vi "Send update actor configuration.vi"(7 "Message Priority (Normal)":T5=enum."Normal", 8 "error in (no error)":errorcluster, 10 "ActorConfiguration":T1={"GlobalConfiguration"={"DeviceFamily"="", "WriteData"=FALSE, "BufferSize_samples"=-1, "SyncDevice"=FALSE, "ExecuteInterruptRoutine"=FALSE, "InterruptRoutineTimeout_ms"=-1}, "DeviceConfiguration"={"DeviceSpecificName"="MIPI_Camera", "HardwareReference"="PXIe-Slot2", "UsedResources"=[{"ResourceLocation"="FrontFacing", "ResourceData"=variant(string "Use this Variant to store your specific resource data.\nThis will be read from and written to with the JSON parsing API.\nIn the child implementation you can use the acessors provided to convert from the specific cluster to your own device's implementation")}]}}, 11 "Message Enqueuer":refnum<class "Message Enqueuer.lvclass">) -> (0 "error out":errorcluster, 3 "Message Enqueuer out":refnum<class "Message Enqueuer.lvclass">)   [LabVIEW 2020, in "Template.lvlib" / "update actor configuration Msg.lvclass"]
doc: "This VI sends the message to an actor."
uses:
  update actor configuration Msg.lvclass
  <vilib>/ActorFramework/Message Enqueuer/Message Enqueuer.lvclass
  <vilib>/ActorFramework/Message Enqueuer/Message Priority.ctl
  template/typedefs/actor configuration.ctl
  template/typedefs/shared actor configuration.ctl
  template/typedefs/resource config/device configuration cluster.ctl
  template/typedefs/resource config/single resource cluster.ctl
  C:/Program Files/National Instruments/LabVIEW 2020/vi.lib/ActorFramework/Message/Message.lvclass
  update actor configuration Msg.lvclass/update actor configuration Msg.ctl
  <vilib>/ActorFramework/Message Enqueuer/Message Enqueuer.lvclass/Message Enqueuer.ctl
  <vilib>/ActorFramework/Message Priority Queue/Priority Enqueue.vi
  template/Template.lvclass
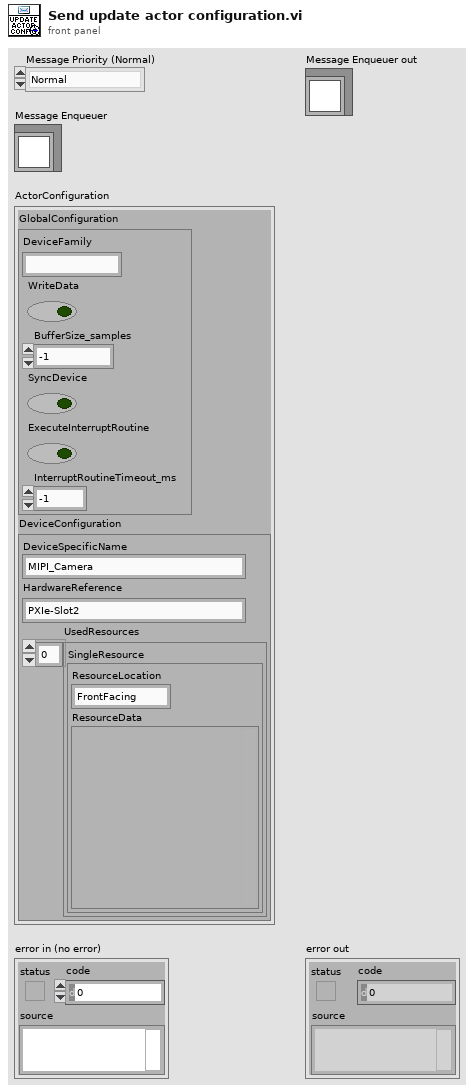
[diagram p1: front panel]
types:
  T1 = typedef "Template.lvlib/Template.lvclass/actor configuration.ctl" = cluster{"GlobalConfiguration":T2, "DeviceConfiguration":T3}
  T2 = typedef "Template.lvlib/Template.lvclass/shared actor configuration.ctl" = cluster{"DeviceFamily":string, "WriteData":bool, "BufferSize_samples":i32, "SyncDevice":bool, "ExecuteInterruptRoutine":bool, "InterruptRoutineTimeout_ms":i32}
  T3 = typedef "Template.lvlib/Template.lvclass/device configuration cluster.ctl" = cluster{"DeviceSpecificName":string, "HardwareReference":string, "UsedResources":T4[]}
  T4 = typedef "Template.lvlib/Template.lvclass/single resource cluster.ctl" = cluster{"ResourceLocation":string, "ResourceData":variant}
  T5 = typedef "Actor Framework.lvlib/Message Enqueuer.lvclass/Message Priority.ctl" = enum16{"Low", "Normal", "High"}
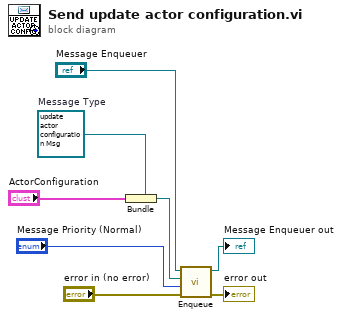
[diagram p0: block diagram]
diagram:
  w2 = refnum<class "update actor configuration Msg.lvclass"> refnum  # Message Type
  n1 = Bundle(cluster=w2, "ActorConfiguration") -> (w3:refnum<class "update actor configuration Msg.lvclass">)
  n2 = call <vilib>:"Enqueue.vi"("error in (no error)"="error in (no error)", "Message Priority (Normal)"="Message Priority (Normal)", "Message"=w3, "Message Enqueuer in"="Message Enqueuer") -> ("error out"=→"error out":errorcluster, "Message Enqueuer out"=→"Message Enqueuer out":refnum<class "Message Enqueuer.lvclass">)  [unwired: 6 in]
